vi "Figure.vi"() -> (27 "error out":errorcluster)   [LabVIEW 2021]
uses:
  <vilib>/vision/Measure.llb/Edge Options.ctl
  <vilib>/vision/Measure.llb/Edge Polarity.ctl
  <vilib>/vision/Measure.llb/Straight Edge Options.ctl
  <vilib>/vision/Measure.llb/Straight Edge Process.ctl
  <vilib>/userDefined/High Color/IMAQdx.ctl
  <vilib>/vision/NI_Vision_Development_Module.lvlib
  <vilib>/vision/driver/NI_Vision_Acquisition_Software.lvlib
panel:
  out "원소":enum16{"원", "정사각형", "직사각형"}(ring)
  out "Distance (calibrated) 2":sgl format="%.2f"
  out "Distance (calibrated)":sgl format="%.2f"
  in  "error in 2":errorcluster
  in  "열거형 2":enum16{"카메라", "파일"}(ring)
  in  "Parameters (Caliper 1)":T1(array[cluster])=[{"Feature"=4, "Points IDs"=[{"GUID"="Find Straight Edge 4", "Index"=0}, {"GUID"="Find Straight Edge 4", "Index"=2}]}] {"Feature" items=["Distance", "Mid Point", "Perpendicular Projection", "Lines Intersection", "Angle from Horizontal", "Angle from Vertical", "Angle Defined by 3 Points", "Angle Defined by 4 Points", "Bissecting Line", "Mid Line", "Center of Mass", "Area", "Line Fit", "Circle Fit", "Ellipse Fit"]}
  in  "Fit Options (Find Straight Edge 4)":T2={"Number of Lines"=1, "Type"=enum."First Edge Rake", "Min. Score"=10.0, "Max. Score"=1000.0, "Orientation"=0.0, "Angle Range"=45.0, "Angle Tolerance"=1.0, "Step Size"=105, "Min. SNR (db)"=0.0, "Min. Points (%)"=25.0, "Hough Iterations"=5} {"Min. Points (%)" min=0.0 max=100.0; "Min. SNR (db)" min=0.0; "Max. Score" min=0.0 max=1024.0; "Min. Score" min=0.0 max=1024.0 step=1.0}
  in  "Options (Find Straight Edge 4)":T6={"Search Direction"=3, "Edge Options"={"Edge Polarity"=0, "Kernel Size"=3, "Width"=3, "Minimum Edge Strength"=10.0, "Interpolation Type"=enum."Bilinear Fixed", "Data Processing Method"=enum."Average"}, "Show Search Area"=TRUE, "Show Search Lines"=TRUE, "Show Edges Found"=TRUE, "Show Result"=TRUE, "Search Area Color"=65280, "Search Lines Color"=255, "Edge Locations Color"=16776960, "Result Color"=16711680, "Overlay Group Name"=""} {"Search Direction" items=["Left to Right", "Right to Left", "Top to Bottom", "Bottom to Top"]; "Edge Options"."Edge Polarity" items=["All Edges", "Rising Edges", "Falling Edges"]; "Edge Options"."Minimum Edge Strength" format="%.2f"; "Edge Options"."Width" step=2; "Edge Options"."Kernel Size" step=2}
  out "Image Out 2":T7(plugin-control)
  in  "Maintain Size (Geometry 1)":bool=TRUE
  out "Image Out":T7(plugin-control)
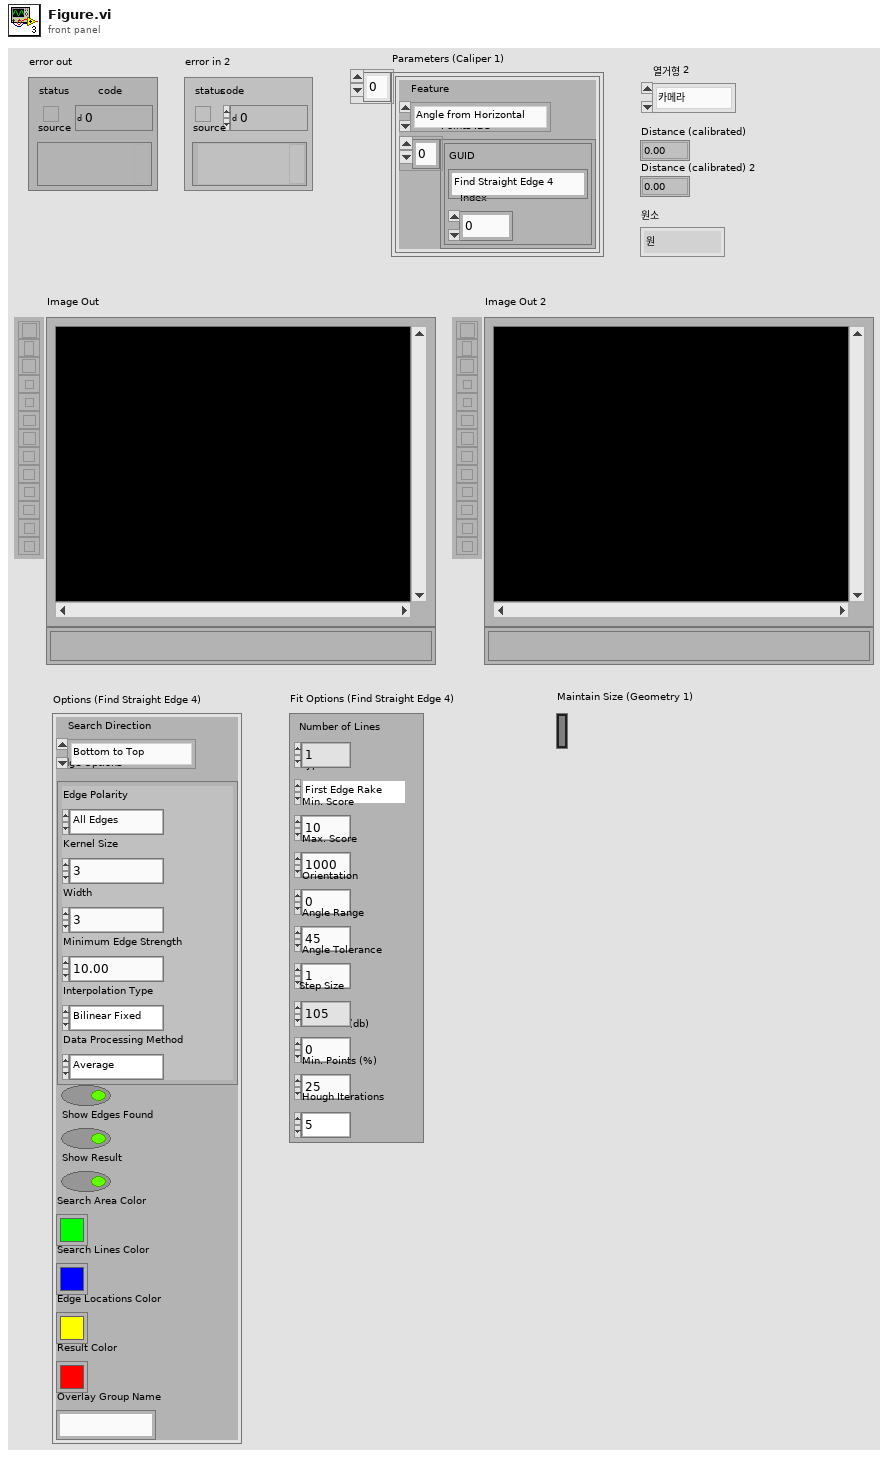
[diagram p1: front panel]
types:
  T1 = cluster{"Feature":u32, "Points IDs":cluster{"GUID":string, "Index":i32}[]}[]
  T2 = typedef "Straight Edge Options.ctl" = cluster{"Number of Lines":i32, "Type":T3, "Min. Score":dbl, "Max. Score":dbl, "Orientation":dbl, "Angle Range":dbl, "Angle Tolerance":dbl, "Step Size":u32, "Min. SNR (db)":dbl, "Min. Points (%)":dbl, "Hough Iterations":i32}
  T3 = typedef "Straight Edge Process.ctl" = enum32{"First Edge Rake", "Best Edge Rake", "Hough Edge Rake", "First Edge Projection", "Best Edge Projection"}
  T4 = typedef "Edge Options.ctl" = cluster{"Edge Polarity":T5, "Kernel Size":u32, "Width":u32, "Minimum Edge Strength":sgl, "Interpolation Type":enum32{"Zero Order", "Bilinear", "Quadratic", "Cubic", "Bilinear Fixed"}, "Data Processing Method":enum32{"Average", "Median"}}
  T5 = typedef "Edge Polarity.ctl" = u32
  T6 = cluster{"Search Direction":u32, "Edge Options":T4, "Show Search Area":bool, "Show Search Lines":bool, "Show Edges Found":bool, "Show Result":bool, "Search Area Color":u32, "Search Lines Color":u32, "Edge Locations Color":u32, "Result Color":u32, "Overlay Group Name":string}
  T7 = typedef "IMAQ Image.ctl" = refnum<image>
  T8 = cluster{"Global Rectangle":i32[], "Contours":cluster{"ID":enum32{"External", "Internal"}, "Type":u32, "Coordinates":i32[]}[]}
  T9 = typedef "Image Type" = u32
  T10 = typedef "IMAQdx.ctl" = refnum<k21>
  T11 = cluster{"Point1 (Pixels)":cluster{"X":sgl, "Y":sgl}, "Point2 (Pixels)":cluster{"X":sgl, "Y":sgl}, "Point1 (Real-World)":cluster{"X":sgl, "Y":sgl}, "Point2 (Real-World)":cluster{"X":sgl, "Y":sgl}, "Angle (Pixel)":dbl, "Angle (Real-World)":dbl, "Score":dbl, "Straightness":dbl, "Average SNR (db)":dbl, "Calibration Valid":bool}[]
  T12 = cluster{"Point1 (Pixels)":cluster{"X":sgl, "Y":sgl}, "Point2 (Pixels)":cluster{"X":sgl, "Y":sgl}, "Point1 (Real-World)":cluster{"X":sgl, "Y":sgl}, "Point2 (Real-World)":cluster{"X":sgl, "Y":sgl}, "Angle (Pixel)":dbl, "Angle (Real-World)":dbl, "Score":dbl, "Straightness":dbl, "Average SNR (db)":dbl, "Calibration Valid":bool}
  T13 = cluster{"Contrast":i32, "Filter width":i32, "Steepness":i32, "Subsampling Ratio":u32, "Show Search Area":bool, "Show Search Lines":bool, "Show Edges Found":bool, "Show Result":bool}
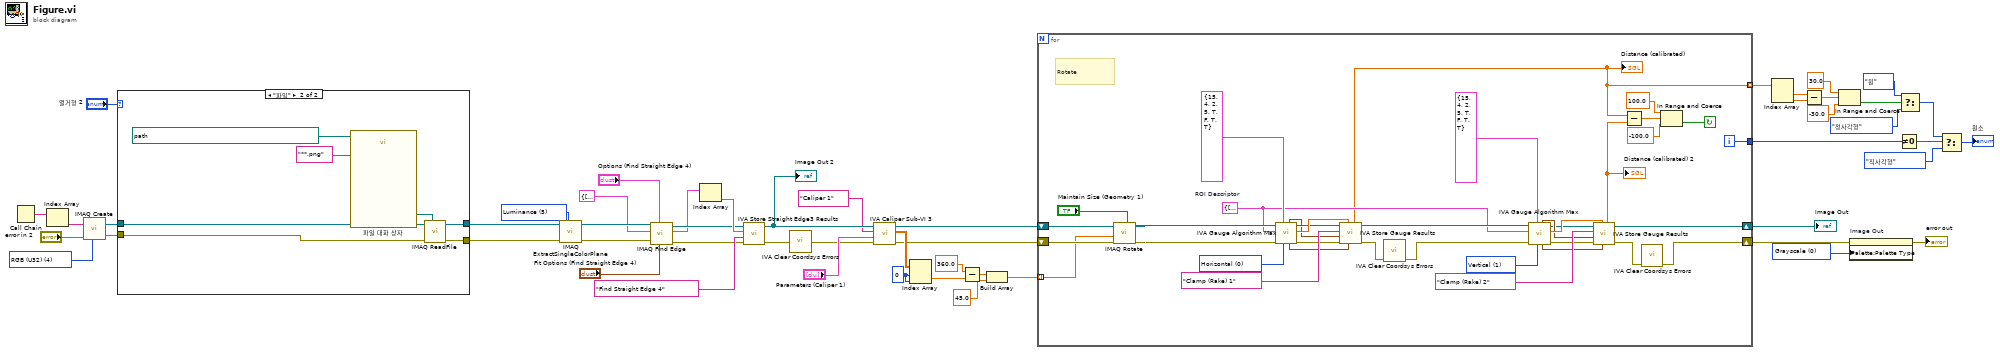
[diagram p0: block diagram]
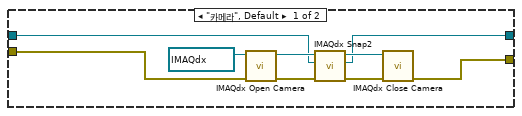
[diagram p2: hidden frame]
diagram:
  w28 = 0 ("인덱스 (행)")
  w31 = T9 4 items=["Grayscale (U8)", "Grayscale (I16)", "Grayscale (SGL)", "Complex (CSG)", "RGB (U32)", "HSL (U32)", "RGB (U64)", "Grayscale (U16)"] ("Image Type")
  w47 = 5 items=["Red", "Green", "Blue", "Hue", "Saturation", "Luminance", "Value", "Intensity"] ("Color Plane (Color Plane Extraction 1)")
  w49 = u32 0 items=["Grayscale", "Binary", "Gradient", "Rainbow", "Temperature", "User Defined", "Binary 16 Bit", "Gradient 16 Bit", "Rainbow 16 Bit", "Temperature 16 Bit", "User Defined 16 Bit"] ("Palette Type")
  n1 = Call Chain() -> (call chain=w33:string[])
  n2 = Index Array(array=w33) -> (element=w34:string)  [unwired: 1 in]
  n3 = call "IMAQ Create"("Image Name"=w34, "Image Type"=w31, "error in (no error)"="error in 2") -> ("New Image"=w30:T7, "error out"=w17:errorcluster)  [unwired: 1 in, 1 out]
  n4 = case shown="\"파일\"" "열거형 2" {
    tunnel: [w53 w67] -> w48
    tunnel: [w54 w66] -> w46
    tunnel: w30 -> [w55 w65]
    tunnel: w17 -> [w52 w64]
    frame "카메라", Default {
      n5 = call <vilib>:"IMAQdx Open Camera.vi"("error in"=w52, "Session In"=T10 "cam7") -> ("error out"=w58:errorcluster, "Session Out"=w59:T10)  [unwired: 8 in]
      n6 = call <vilib>:"IMAQdx Snap2.vi"("error in"=w58, "Image In"=w55, "Session In"=w59) -> ("error out"=w56:errorcluster, "Image Out"=w54:T7, "Session Out"=w57:T10)  [unwired: 6 in]
      n7 = call <vilib>:"IMAQdx Close Camera.vi"("error in"=w56, "Session In"=w57) -> ("error out"=w53:errorcluster)  [unwired: 9 in]
    }
    frame "파일" {
      n8 = call "파일 대화 상자"("start path"=path "C:/Users/user/Desktop/이미지파일", "pattern (all files)"="**.png") -> ("selected path"=w61:path)  [unwired: 10 in, 3 out]
      n9 = call "IMAQ ReadFile"("File Path"=w61, "error in (no error)"=w64, "Image"=w65) -> ("error out"=w67:errorcluster, "Image Out"=w66:T7)  [unwired: 2 in, 5 out]
    }
  }
  n10 = call "IMAQ ExtractSingleColorPlane"("Color Plane"=w47, "error in (no error)"=w48, "Image Src"=w46) -> ("error out"=w45:errorcluster, "Image Dst Out"=w44:T7)  [unwired: 1 in, 6 out]
  n11 = call "IMAQ Find Edge"("Line Fit Options"="Fit Options (Find Straight Edge 4)", "Options"="Options (Find Straight Edge 4)", "error in (no error)"=w45, "ROI Descriptor"=T8 {"Global Rectangle"=[66, 463, 1114, 860], "Contours"=[{"ID"=enum."External", "Type"=12, "Coordinates"=[66, 463, 1114, 860, 0]}]} ("ROI Descriptor (Find Straight Edge 4)"), "Image"=w44) -> ("error out"=w37:errorcluster, "Straight Edges"=w36:T11, "Image Out"=w38:T7)  [unwired: 1 in, 3 out]
  n12 = Index Array(array=w36) -> (element=w39:T12)  [unwired: 1 in]
  n13 = call <vilib>:"IVA Store Straight Edge3 Results.vi"("error in (no error)"=w37, "Step Name"="Find Straight Edge 4", "Straight Edge"=w39, "Image in"=w38) -> ("error out"=w18:errorcluster, "Image dup"=w21:T7)  [unwired: 1 in, 5 out]
  "Image Out 2" <- w21
  n14 = call <vilib>:"IVA Clear Coordsys Errors.vi"("error in (no error)"=w18) -> ()  [unwired: 10 in, 1 out]
  n15 = call <vilib>:"IVA Caliper Sub-VI 3.vi"("error in"=w18, "Parameters"="Parameters (Caliper 1)", "Step Name"="Caliper 1", "Image In"=w21) -> ("error out"=w22:errorcluster, "Results (Pixels)"=w29:sgl[][], "Image Out"=w23:T7)  [unwired: 1 in, 4 out]
  n16 = Index Array(array=w29, index (row)=w28, index (col)=w28) -> (element=w26:sgl)
  n17 = Subtract(x=sgl 360.0, y=w26) -> (x-y=w25:sgl)
  n18 = Build Array(w25, sgl 45.0 ("원소")) -> (w2:sgl[])
  n19 = for {
    shift-right: [w84] -> w51
    shift-left: w22 -> [w95]
    shift-right: [w73] -> w1
    shift-left: w23 -> [w94]
    tunnel: [w72] -> w16 mode=indexing
    tunnel: [w71] -> w9
    tunnel: w2 -> [w70] mode=indexing
    i -> [w71]
    stop <- w74 continue-if-true
    w89 = u32 1 items=["Horizontal", "Vertical"] ("Scanning axis")
    w102 = u32 0 items=["Horizontal", "Vertical"] ("Scanning axis")
    w82 = T8 {"Global Rectangle"=[300, 200, 1000, 788], "Contours"=[{"ID"=enum."External", "Type"=12, "Coordinates"=[300, 200, 1000, 788, 0]}]}  # ROI Descriptor
    # "Rotate"
    n20 = call "IMAQ Rotate"("Maintain Size"="Maintain Size (Geometry 1)", "error in (no error)"=w95, "Angle (degrees)"=w70, "Image Src"=w94) -> ("error out"=w96:errorcluster, "Image Dst Out"=w93:T7)  [unwired: 6 in]
    n21 = call <vilib>:"IVA Gauge Algorithm Max.vi"("Scanning axis"=w102, "Settings"=T13 {"Contrast"=15, "Filter width"=4, "Steepness"=2, "Subsampling Ratio"=5, "Show Search Area"=TRUE, "Show Search Lines"=FALSE, "Show Edges Found"=TRUE, "Show Result"=TRUE}, "error in (no error)"=w96, "ROI Descriptor"=w82, "Image"=w93) -> ("error out"=w97:errorcluster, "Distance"=w101:sgl, "Image Out"=w98:T7, "Distance Points"=w80:cluster{"X":sgl, "Y":sgl}[], "Points of Contact"=w81:cluster{"X":sgl, "Y":sgl}[])  [unwired: 1 in, 1 out]
    n22 = call <vilib>:"IVA Store Gauge Results.vi"("Distance Points"=w80, "Distance"=w101, "error in (no error)"=w97, "Points of Contact"=w81, "Step Name"="Clamp (Rake) 1", "Image in"=w98) -> ("error out"=w99:errorcluster, "Image dup"=w83:T7, "Distance (calibrated)"=w72:sgl)  [unwired: 3 out]
    "Distance (calibrated)" <- w72
    n23 = call <vilib>:"IVA Clear Coordsys Errors.vi"("error in (no error)"=w99) -> ("error out"=w87:errorcluster)  [unwired: 10 in]
    n24 = call <vilib>:"IVA Gauge Algorithm Max.vi"("Scanning axis"=w89, "Settings"=T13 {"Contrast"=15, "Filter width"=4, "Steepness"=2, "Subsampling Ratio"=5, "Show Search Area"=TRUE, "Show Search Lines"=FALSE, "Show Edges Found"=TRUE, "Show Result"=TRUE}, "error in (no error)"=w87, "ROI Descriptor"=w82, "Image"=w83) -> ("error out"=w86:errorcluster, "Distance"=w90:sgl, "Image Out"=w69:T7, "Distance Points"=w68:cluster{"X":sgl, "Y":sgl}[], "Points of Contact"=w79:cluster{"X":sgl, "Y":sgl}[])  [unwired: 1 in, 1 out]
    n25 = call <vilib>:"IVA Store Gauge Results.vi"("Distance Points"=w68, "Distance"=w90, "error in (no error)"=w86, "Points of Contact"=w79, "Step Name"="Clamp (Rake) 2", "Image in"=w69) -> ("error out"=w85:errorcluster, "Image dup"=w73:T7, "Distance (calibrated)"=w78:sgl)  [unwired: 3 out]
    "Distance (calibrated) 2" <- w78
    n26 = Subtract(x=w72, y=w78) -> (x-y=w77:sgl)
    n27 = call <vilib>:"IVA Clear Coordsys Errors.vi"("error in (no error)"=w85) -> ("error out"=w84:errorcluster)  [unwired: 10 in]
    n28 = In Range and Coerce(upper limit=sgl 100.0 ("상위 리미트"), x=w77, lower limit=sgl -100.0 ("하위 리미트")) -> (In Range?=w74:bool)  [unwired: 1 out]
  }
  "Image Out" <- w1
  n29 = Index Array(array=w16) -> (element #1=w15:sgl, element #2=w14:sgl)  [unwired: 2 in]
  n30 = Subtract(x=w15, y=w14) -> (x-y=w13:sgl)
  n31 = In Range and Coerce(upper limit=sgl 30.0 ("상위 리미트"), x=w13, lower limit=sgl -30.0 ("하위 리미트")) -> (In Range?=w10:bool)  [unwired: 1 out]
  n32 = property on="Image Out" class="ImageControl"(error in=w51, "Palette:Palette Type"=w49) -> (error out=→"error out":errorcluster)  [unwired: 1 in, 1 out]
  n33 = Not Equal To 0?(x=w9) -> (x != 0?=w4:bool)
  n34 = Select(t=enum16{"원", "정사각형", "직사각형"}."원", s=w10, f=enum16{"원", "정사각형", "직사각형"}."정사각형") -> (s? t:f=w8:enum16{"원", "정사각형", "직사각형"})
  n35 = Select(t=w8, s=w4, f=enum16{"원", "정사각형", "직사각형"}."직사각형") -> (s? t:f=→"원소":enum16{"원", "정사각형", "직사각형"})
